vi "Set Boolean Button Text.vi"(10 "text":string="thisIsAtext", 11 "boolean ref in":refnum<vi>) -> (3 "bool ref out":refnum<vi>)   [LabVIEW 2020, in "FrameEditor.lvlib"]
uses:
  FrameEditor.lvlib
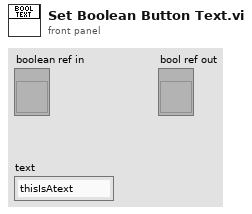
[diagram p1: front panel]
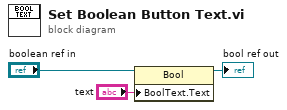
[diagram p0: block diagram]
diagram:
  n1 = property class="Bool"(reference="boolean ref in", "BoolText.Text"="text") -> (reference out=→"bool ref out":refnum<vi>)  [unwired: 1 in, 1 out]
